vi "Constants.vi"() -> ()   [LabVIEW 2018]
panel:
  out "Max Velocity (Raw Units)":dbl=2255.0
  out "F for Motion Magic":dbl=0.453658
  out "railEndPosition (Inches)":dbl
  out "railBeginPosition (Inches)":dbl
  out "railEndPosition":dbl=20000.0
  out "railBeginPosition":dbl=500.0
  out "trueRailMaxPosition (Raw Units)":dbl=20610.0
  out "trueRailBeginPosition (Raw Units)":dbl
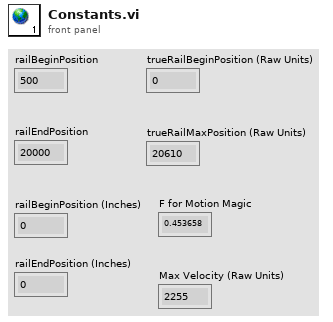
[diagram p1: front panel]
diagram:
